vi "Build API URL.vi"(8 "error in (no error)":errorcluster, 10 "API Endpoint":T1, 11 "GCentral API in":refnum<class "GCentral API.lvclass">) -> (0 "error out":errorcluster, 2 "URL":string, 3 "GCentral API out":refnum<class "GCentral API.lvclass">)   [LabVIEW 2020, in "GCentral-API.lvlib" / "GCentral API.lvclass"]
uses:
  GCentral API.lvclass
  API Endpoint.ctl
  GCentral API.lvclass/GCentral API.ctl
  GCentral-API.lvlib
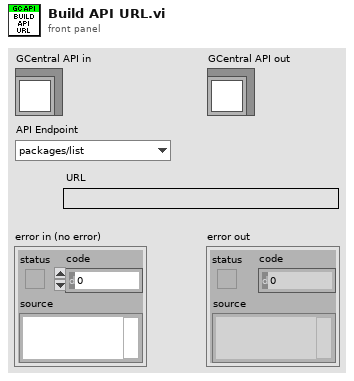
[diagram p1: front panel]
types:
  T1 = typedef "GCentral-API.lvlib/API Endpoint.ctl" = enum16{"packages/list", "packages/search"}
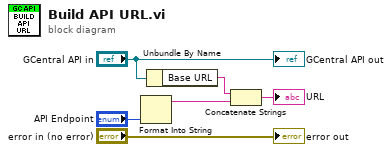
[diagram p0: block diagram]
diagram:
  n1 = Format Into String("API Endpoint") -> (resulting string=w3:string)  [unwired: 3 in, 1 out]
  n2 = Unbundle By Name("GCentral API in") -> ("Base URL"=w2:string)
  n3 = Concatenate Strings(w2, w3) -> (→"URL":string)
  "error out" <- "error in (no error)"
  "GCentral API out" <- "GCentral API in"
